vi "OMV_Txbuffer.vi"(8 "error in (no error)":errorcluster, 11 "VISA Refnum in":refnum<visa-resource-name>) -> (0 "error out":errorcluster, 2 "Data":dbl, 3 "VISA Refnum out":refnum<visa-resource-name>)   [LabVIEW 2017]
panel:
  out "Tx Buffer":string
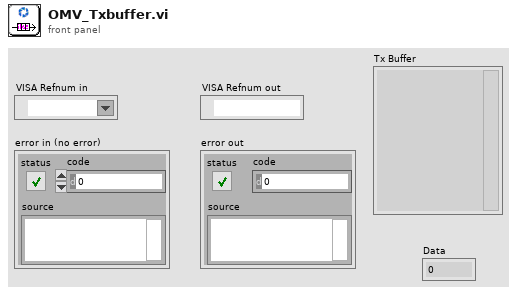
[diagram p1: front panel]
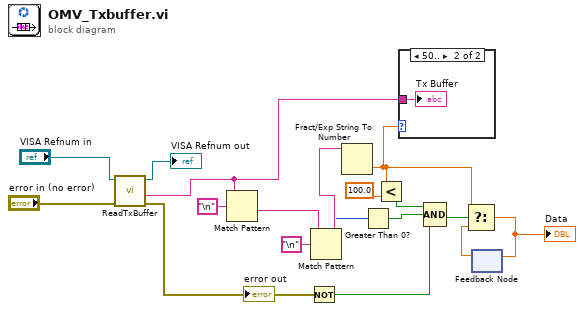
[diagram p0: block diagram]
diagram:
  n1 = call "ReadTxBuffer.vi"("error in"="error in (no error)", "VISA Refnum in"="VISA Refnum in") -> ("error out"=w2:errorcluster, "Tx Buffer"=w7:string, "VISA Refnum out"=→"VISA Refnum out":refnum<visa-resource-name>)  [unwired: 6 in, 1 out]
  "error out" <- w2
  n2 = Match Pattern(string=w7, regular expression="\n") -> (after substring=w5:string)  [unwired: 1 in, 3 out]
  n3 = Not(x=w2) -> (.not. x?=w1:bool)
  n4 = Match Pattern(string=w5, regular expression="\n") -> (before substring=w4:string, offset past match=w3:i32)  [unwired: 1 in, 2 out]
  n5 = Fract/Exp String To Number(string=w4) -> (number=w8:dbl)  [unwired: 3 in, 1 out]
  n6 = Greater Than 0?(x=w3) -> (x > 0?=w10:bool)
  n7 = Less?(x=w8, y=100.0) -> (x < y?=w11:bool)
  n8 = case shown="50.." w8 {
    tunnel: w7 -> [_ w19]
    frame 0, Default {
    }
    frame 50.. {
      "Tx Buffer" <- w19
    }
  }
  n9 = Compound Arithmetic op=AND(w11, w10, w1) -> (w9:bool)
  n10 = feedback #1() -> (w14:dbl)  [unwired: 1 in]
  n11 = Select(t=w8, s=w9, f=w14) -> (s? t:f=w13:dbl)
  "Data" <- w13
  n12 = feedback-in #1(w13) -> ()
